vi "Ctor.vi"(8 "error in (no error)":errorcluster, 10 "Server TCP Port":u16=4763, 11 "Server Address":string="127.0.0.1") -> (0 "error out":errorcluster, 3 "LV Client out":refnum<class "LV Client.lvclass">)   [LabVIEW 2020, in "LV Client.lvclass"]
uses:
  LV Client.lvclass
  LV Client.lvclass/LV Client.ctl
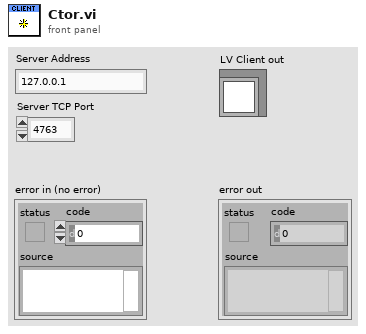
[diagram p1: front panel]
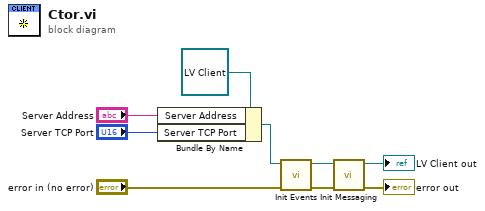
[diagram p0: block diagram]
diagram:
  n1 = Bundle By Name(cluster=refnum<class "LV Client.lvclass"> refnum ("LV Client in"), "Server Address"="Server Address", "Server TCP Port"="Server TCP Port") -> (w5:refnum<class "LV Client.lvclass">)
  n2 = call "Init Events.vi"("error in (no error)"="error in (no error)", "LV Client in"=w5) -> ("error out"=w3:errorcluster, "LV Client out"=w4:refnum<class "LV Client.lvclass">)  [unwired: 8 in]
  n3 = call "Init Messaging.vi"("error in (no error)"=w3, "LV Client in"=w4) -> ("error out"=→"error out":errorcluster, "LV Client out"=→"LV Client out":refnum<class "LV Client.lvclass">)  [unwired: 8 in]
